vi "libcall.vi"(8 "error in (no error)":errorcluster, 9 "Parameter":string, 10 "Function":string, 11 "input":i32) -> (0 "error out":errorcluster, 2 "id":string)   [LabVIEW 2015]
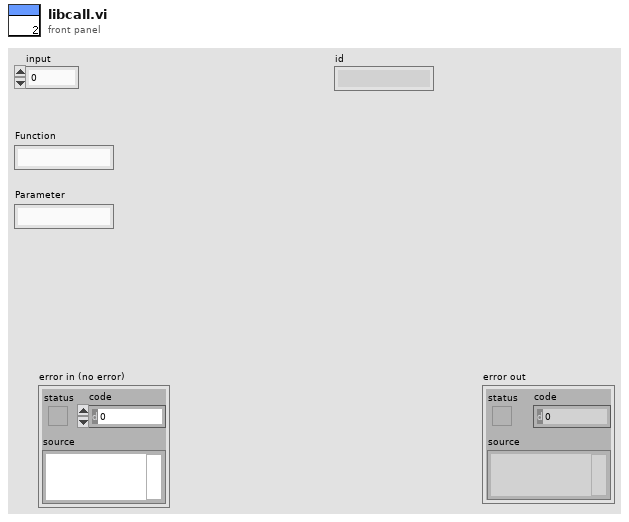
[diagram p1: front panel]
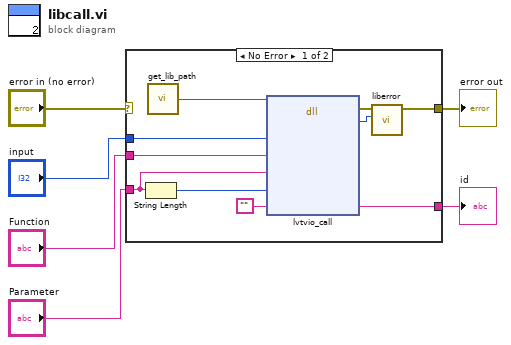
[diagram p0: block diagram]
diagram:
  n1 = case shown="No Error" "error in (no error)" {
    selector: "error in (no error)" -> [_ w17]
    tunnel: [w7 w17] -> w5
    tunnel: "Function" -> [w15 _]
    tunnel: "Parameter" -> [w11 _]
    tunnel: [w13 _] -> w2
    tunnel: "input" -> [w10 _]
    frame No Error {
      n2 = String Length(string=w11) -> (length=w12:i32)
      n3 = call "get_lib_path.vi"() -> ("Path"=w16:path)
      n4 = dll-call lib="C:/GoProgramming/src/github.com/joernweissenborn/thingiverseio/build/libthingiverse.dll" fn="lvtvio_call"(path in=w16, "input"=w10, "function"=w15, "params"=w11, "params_size"=w12, "id"="") -> (error out=w8:errorcluster, "return type"=w9:i32, "id"=w13:string)  [unwired: 6 in, 1 out]
      n5 = call "liberror.vi"("tvio errors"=w9, "error in (no error)"=w8) -> ("error out"=w7:errorcluster)  [unwired: 9 in]
    }
    frame Error {
    }
  }
  "error out" <- w5
  "id" <- w2
